vi "Create.vi"(8 "Error In":errorcluster) -> (0 "Error Out":errorcluster)   [LabVIEW 2016, in "Anti-Spam Tester (AST).lvlib" / "AST MHL Queue.lvclass"]
doc: "Creates the module's command queue. This queue is used to issue commands (or requests) to the module. The queue size is -1 (unlimited).\n\nThis VI raises an error if a queue of the same name already exists. For example, this can happen if the 'Create' VI is called twice in a row, or called twice without 'Destroy' having been called in between.\n\nRecommended use: Call 'Create' only once during the lifetime of the app. Call it as part of the module init routine (before MHL)."
uses:
  AST MHL Queue.lvclass
  Message (cluster).ctl
  Command (enum).ctl
  Queue Reference (library variable).vi
  Anti-Spam Tester (AST).lvlib
panel:
  # "Input\nInputs to the VI"
  # "Development\nControls or indicators that are useful for development or testing, but which are not outputs of the VI."
  # "Output\nOutputs of the VI"
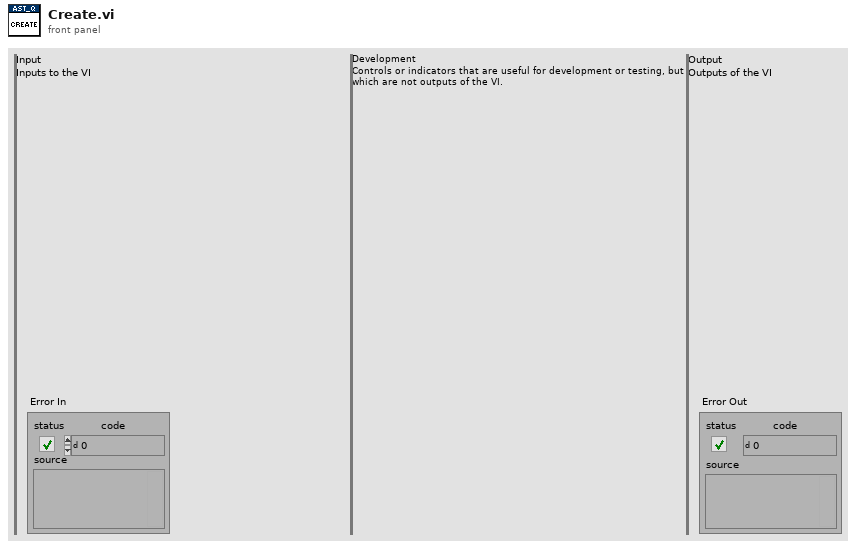
[diagram p1: front panel]
types:
  T1 = typedef "Anti-Spam Tester (AST).lvlib/AST MHL Queue.lvclass/Message (cluster).ctl" = cluster{"Command":T2, "Data":variant}
  T2 = typedef "Anti-Spam Tester (AST).lvlib/AST MHL Queue.lvclass/Command (enum).ctl" = enum16{"Init AST", "Close AST", "Config GUI - Init", "Config GUI - Spamming Has Started", "Config GUI - Spamming Has Stopped", "Spam"}
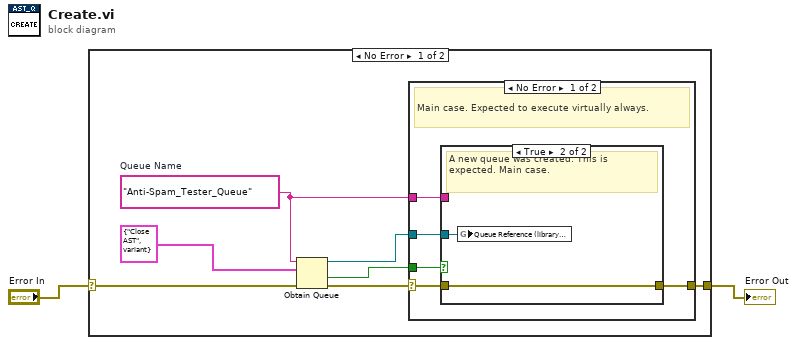
[diagram p0: block diagram]
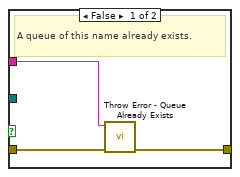
[diagram p2: hidden frame]
diagram:
  n1 = case shown="No Error" "Error In" {
    selector: "Error In" -> [w9 w21]
    tunnel: [w6 w21] -> w1
    frame No Error {
      w4 = "Anti-Spam_Tester_Queue"  # Queue Name
      n2 = Obtain Queue(name (unnamed)=w4, element data type=T1 {"Command"=enum."Close AST", "Data"=variant} ("Queue Message"), error in (no error)=w9) -> (queue out=w3:refnum<queue>, created new?=w5:bool, error out=w7:errorcluster)  [unwired: 2 in]
      n3 = case shown="No Error" w7 {
        selector: w7 -> [w14 w20]
        tunnel: [w13 w20] -> w6
        tunnel: w5 -> [w12 _]
        tunnel: w4 -> [w11 _]
        tunnel: w3 -> [w10 _]
        frame No Error {
          # "Main case. Expected to execute virtually always."
          n4 = case shown="True" w12 {
            tunnel: w14 -> [w17 w19]
            tunnel: [w16 w19] -> w13
            tunnel: w11 -> [w15 _]
            tunnel: w10 -> [_ w18]
            frame False {
              # "A queue of this name already exists."
              n5 = call "Throw Error - Queue Already Exists.vi"(8:w17, 11:w15) -> (0:w16:errorcluster)  [unwired: 9 in]
            }
            frame True {
              # "A new queue was created. This is expected. Main case."
              n6 = global write "Queue Reference (library variable).vi" item#0(w18) -> ()
            }
          }
        }
        frame Error {
          # "Pass the error unaltered."
          # "Error upstream."
        }
      }
    }
    frame Error {
    }
  }
  "Error Out" <- w1
